vi "Initiate and Generate Time (Multi).vi"(0 "niUsrpRio Sessions":T3[](array[typedef]) {"Daughterboard Clock Rate" format="%#.3pHz"; "FPGA Data Clock Rate" format="%#.3pHz"; "Data Clock Rate" format="%#.3pHz"; "Characterization Data"."Frequencies [Hz]" format="%#_6p"; "EEPROM Characterization Header"."Pointer to Device Data Header" format="%x"; "EEPROM Characterization Header"."Checksum" format="%x"; "Device Data Header"."Pointer to Characterization Data" format="%x"; "Device Data Header"."Checksum" format="%x"; "EEPROM Header"."Pointer to User Header" format="%x"; "EEPROM Header"."Pointer to Factory Header" format="%x"; "EEPROM Header"."Product Code" format="%x"; "EEPROM Header"."Checksum" format="%x"}, 1 "tx channels":T2(array[cluster]) {"tx.coerced configurations"."coerced sample rates" format="%#.3pS/s"; "tx.coerced configurations"."coerced levels" format="%#.3gdBm"; "tx.coerced configurations"."coerced lo frequencies" format="%#.3pHz"; "tx.coerced configurations"."coerced frequencies" format="%#.3pHz"; "tx config"."tone frequency" format="%#.3pHz"; "tx config"."sample rate" format="%#.3pS/s"; "tx config"."rf config 0"."level" format="%#_gdBm"; "tx config"."rf config 0"."lo frequency" format="%#.3pHz"; "tx config"."rf config 0"."frequency" format="%#.3pHz"; "tx config"."rf config 1"."level" format="%#_gdBm"; "tx config"."rf config 1"."lo frequency" format="%#.3pHz"; "tx config"."rf config 1"."frequency" format="%#.3pHz"}, 5 "first iteration":bool, 7 "start trigger time":timestamp, 11 "error in":errorcluster) -> (4 "niUsrpRio Sessions (out)":T3[](array[typedef]) {"Daughterboard Clock Rate" format="%#.3pHz"; "FPGA Data Clock Rate" format="%#.3pHz"; "Data Clock Rate" format="%#.3pHz"; "Characterization Data"."Frequencies [Hz]" format="%#_6p"; "EEPROM Characterization Header"."Pointer to Device Data Header" format="%x"; "EEPROM Characterization Header"."Checksum" format="%x"; "Device Data Header"."Pointer to Characterization Data" format="%x"; "Device Data Header"."Checksum" format="%x"; "EEPROM Header"."Pointer to User Header" format="%x"; "EEPROM Header"."Pointer to Factory Header" format="%x"; "EEPROM Header"."Product Code" format="%x"; "EEPROM Header"."Checksum" format="%x"}, 15 "error out":errorcluster)   [LabVIEW 2015]
doc: "Writes baseband waveform to the device then initiates generation.\n\nVIs that must execute before this VI:\nOpen and Configure.vi\n\n<B>Input Parameters</B>\n\n<B>niUsrpRio Session</B> is the object created by the Open VI and used as the session handle for the USRP RIO design library.\n\n<B>first iteration</B> is used to determine if the device needs to be triggered. If this VI is in a loop, wire the iteration count to Equals Zero and then to this terminal. If this VI is not in a loop, wire a TRUE constant to this this terminal.\n\n<B>start trigger time</B> specifies the absolute time to initiate the start trigger. Only applies when the start trigger is set to Future Event.\n\n<B>error in</B> describes error conditions that occur before this node runs. This input provides standard 'error in' functionality.\n\n<B>Output Parameters</B>\n\n<B>niUsrpRio Session (out)</B> is the niUsrpRio session used in all subsequent USRP RIO design library host VIs.\n\n<B>error out</B> contains error information. This output provides standard 'error out' functionality."
uses:
  <instrlib>/niUsrpRio/Config/v1/Host/Public/niUsrpRio Session.ctl
  <instrlib>/_niInstr/Register Bus/v0/Host/Public/Register Bus Session.ctl
  <instrlib>/_niInstr/Register Bus/v0/Host/Private/Session Data.ctl
  <instrlib>/niUsrpRio/Config/v1/Host/Private/DB Queue Reference.ctl
  <instrlib>/niUsrpRio/Config/v1/Host/Private/Daughterboard Data.ctl
  <instrlib>/niUsrpRio/Config/v1/Host/Private/ATR state data.ctl
  <instrlib>/niUsrpRio/Config/v1/Host/Private/Antenna Configuration.ctl
  <instrlib>/niUsrpRio/Config/v1/Host/Private/CPLD Power Mode.ctl
  <instrlib>/niUsrpRio/Config/v1/Host/Public/EEPROM Header.ctl
  <instrlib>/niUsrpRio/Config/v1/Host/Public/EEPROM Device Data Header.ctl
  <instrlib>/niUsrpRio/Config/v1/Host/Public/EEPROM Characterization Header.ctl
  <instrlib>/niUsrpRio/Config/v1/Host/Public/Characterization Data.ctl
  <instrlib>/niUsrpRio/Config/v1/Host/Public/IQ Imbalance.ctl
  Start Trigger.ctl
  Write Tx Data (I16 multi).vi
  <instrlib>/_niInstr/Register Bus/v0/Host/niInstr Register Bus v0 Host.lvlib
  <instrlib>/niUsrpRio/Config/v1/Host/niUsrpRio Config v1 Host.lvlib
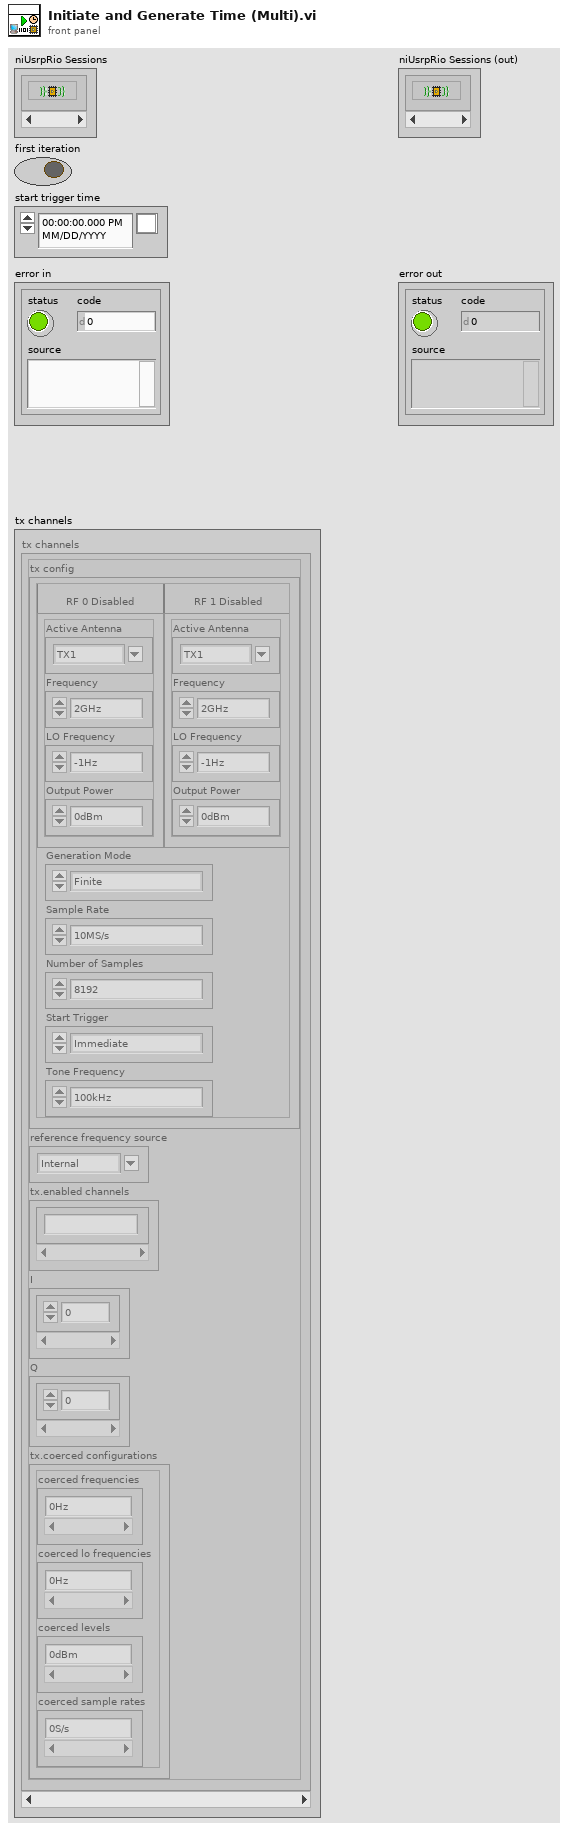
[diagram p1: front panel]
types:
  T1 = typedef "Start Trigger.ctl" = enum8{"Software", "Digital Edge", "Rx Start Trigger", "Tx Start Trigger", "Immediate", "Future Time Event"}
  T2 = cluster{"tx config":cluster{"rf enable 0":bool, "rf config 0":cluster{"antenna":string, "frequency":dbl, "lo frequency":dbl, "level":dbl}, "rf enable 1":bool, "rf config 1":cluster{"antenna":string, "frequency":dbl, "lo frequency":dbl, "level":dbl}, "transfer mode":enum16{"Finite", "Continuous"}, "sample rate":dbl, "number of samples":u32, "start trigger":T1, "tone frequency":dbl}, "reference frequency source":string, "tx.enabled channels":string[], "I":i16[], "Q":i16[], "tx.coerced configurations":cluster{"coerced frequencies":dbl[], "coerced lo frequencies":dbl[], "coerced levels":dbl[], "coerced sample rates":dbl[]}}[]
  T3 = typedef "niUsrpRio Config v1 Host.lvlib/niUsrpRio Session.ctl" = cluster{"FPGA Interface":refnum<k20>, "RIO Interface Number":u32, "Data Clock Rate":u32, "FPGA Data Clock Rate":u32, "Global Settings Register Bus":T4, "Radio 0 Settings Register Bus":T4, "Radio 1 Settings Register Bus":T4, "Radio Settings Bus Semaphore":T5, "DB Queues":T6[], "Characterization Data Valid?":bool, "EEPROM Header":T7, "Device Data Header":T8, "EEPROM Characterization Header":T9, "Characterization Data":T10[], "FPGA Current Version":u32, "FPGA Oldest Compatible Version":u32, "Fixed Logic Current Version":u32, "Fixed Logic Oldest Compatible Version":u32, "FPGA Radio Settings Bus Current Version":u32, "FPGA Radio Settings Bus Oldest Compatible Version":u32, "FPGA Board Config Current Version":u32, "FPGA Board Config Oldest Compatible Version":u32, "Daughterboard Clock Rate":u32}
  T4 = typedef "niInstr Register Bus v0 Host.lvlib/Register Bus Session.ctl" = refnum<queue>
  T5 = typedef "Semaphore RefNum" = refnum<k1>
  T6 = typedef "niUsrpRio Config v1 Host.lvlib/DB Queue Reference.ctl" = refnum<queue>
  T7 = typedef "niUsrpRio Config v1 Host.lvlib/EEPROM Header.ctl" = cluster{"Checksum":u32, "Product Code":u16, "Hardware Current Version":u16, "Hardware Oldest Compatible Version":u16, "EEPROM Map Current Version":u16, "EEPROM Map Oldest Compatible Version":u16, "User Password":string, "Pointer to Factory Header":u32, "Pointer to User Header":u32, "Recommended Interval":u16, "Number of Reserved Bytes":i32, "Number of Daughterboards":u8, "Daughterboard IDs":u16[], "Daughterboard Serial Numbers":string[]}
  T8 = typedef "niUsrpRio Config v1 Host.lvlib/EEPROM Device Data Header.ctl" = cluster{"Checksum":u32, "Number of Channels":u8, "Number of Gain Settings":u16[], "Pointer to Characterization Data":u32[], "Number of Reserved Bytes":i32, "Number of Frequencies":u16[]}
  T9 = typedef "niUsrpRio Config v1 Host.lvlib/EEPROM Characterization Header.ctl" = cluster{"Checksum":u32, "Date":timestamp, "Temperature":sgl, "Misc. Info":string, "Pointer to Device Data Header":u32, "Number of Reserved Bytes":i32}
  T10 = typedef "niUsrpRio Config v1 Host.lvlib/Characterization Data.ctl" = cluster{"Gains[dB]":dbl[], "Frequencies [Hz]":dbl[], "IQ Imbalance Table":T11[], "Measured Gains[dB]":dbl[][]}
  T11 = typedef "niUsrpRio Config v1 Host.lvlib/IQ Imbalance.ctl" = cluster{"Gain Imbalance [linear]":dbl, "Phase Imbalance [radians]":dbl, "Offset":cdb}
  T12 = cluster{"tx config":cluster{"rf enable 0":bool, "rf config 0":cluster{"antenna":string, "frequency":dbl, "lo frequency":dbl, "level":dbl}, "rf enable 1":bool, "rf config 1":cluster{"antenna":string, "frequency":dbl, "lo frequency":dbl, "level":dbl}, "transfer mode":enum16{"Finite", "Continuous"}, "sample rate":dbl, "number of samples":u32, "start trigger":T1, "tone frequency":dbl}, "reference frequency source":string, "tx.enabled channels":string[], "I":i16[], "Q":i16[], "tx.coerced configurations":cluster{"coerced frequencies":dbl[], "coerced lo frequencies":dbl[], "coerced levels":dbl[], "coerced sample rates":dbl[]}}
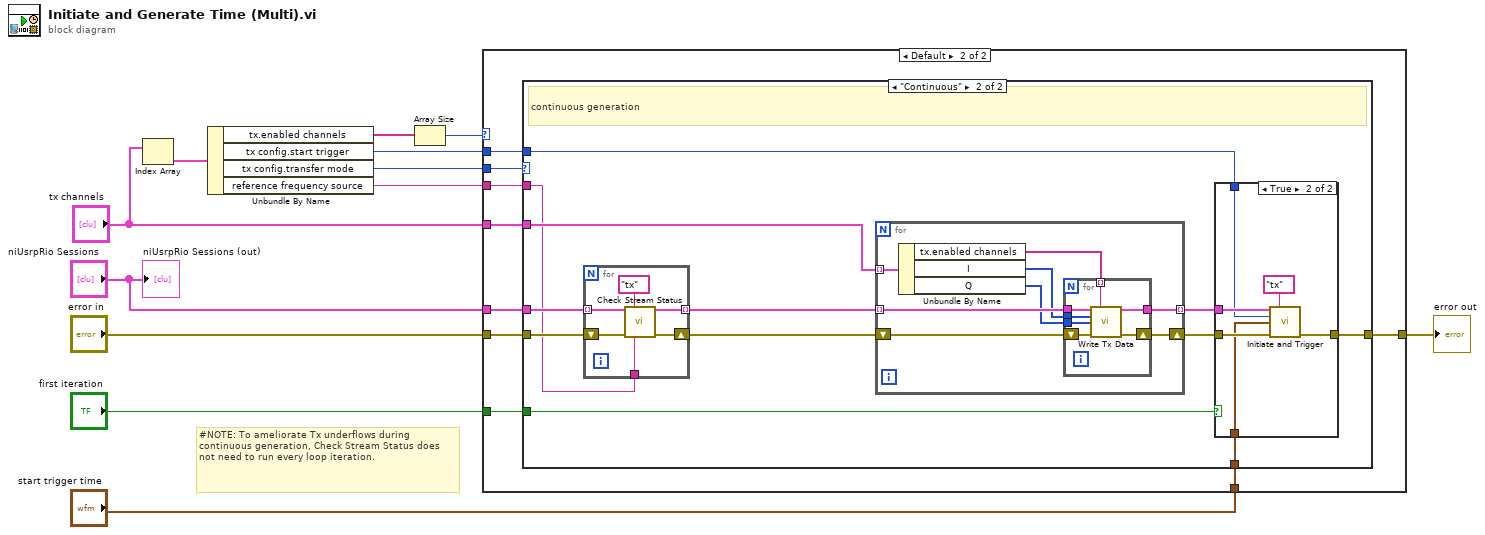
[diagram p0: block diagram]
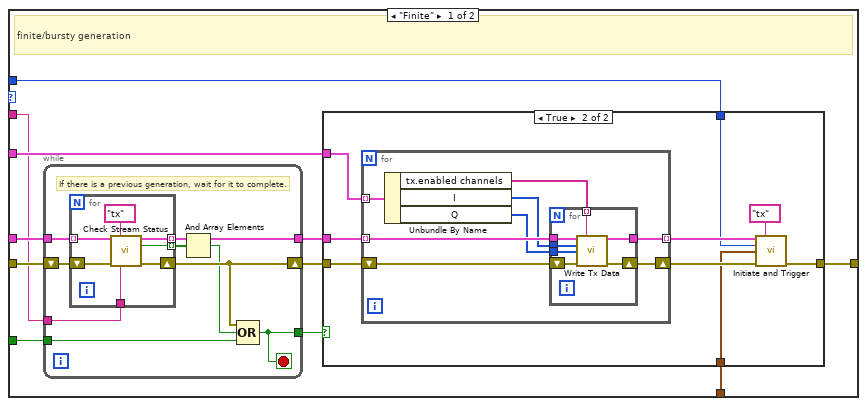
[diagram p3: hidden frame]
diagram:
  # "#NOTE: To ameliorate Tx underflows during continuous generation, Check Stream Status does not need to run every loop iteration."
  n1 = Index Array(array="tx channels") -> (element=w9:T12)  [unwired: 1 in]
  n2 = Unbundle By Name(w9) -> ("tx.enabled channels"=w5:string[], "tx config.start trigger"=w6:T1, "tx config.transfer mode"=w10:enum16{"Finite", "Continuous"}, "reference frequency source"=w7:string)
  n3 = Array Size(array=w5) -> (size(s)=w4:i32)
  n4 = case shown="Default" w4 {
    tunnel: "niUsrpRio Sessions" -> [_ w22]
    tunnel: "error in" -> [w13 w21]
    tunnel: [w13 w20] -> w11
    tunnel: "first iteration" -> [_ w16]
    tunnel: w10 -> [_ w19]
    tunnel: "tx channels" -> [_ w18]
    tunnel: w7 -> [_ w14]
    tunnel: w6 -> [_ w17]
    tunnel: "start trigger time" -> [_ w15]
    frame 0 {
      # "do nothing if there are zero enabled channels"
    }
    frame Default {
      n5 = case shown="\"Continuous\"" w19 {
        tunnel: w22 -> [w24 w79]
        tunnel: w21 -> [w25 w78]
        tunnel: [w33 w86] -> w20
        tunnel: w18 -> [w32 w85]
        tunnel: w17 -> [w31 w84]
        tunnel: w16 -> [w30 w81]
        tunnel: w14 -> [w23 w75]
        tunnel: w15 -> [w28 w80]
        frame "Finite" {
          # "finite/bursty generation"
          n6 = while {
            tunnel: w23 -> [w36]
            shift-right: [w42] -> w27
            shift-left: w25 -> [w39]
            tunnel: w30 -> [w41]
            tunnel: [w34] -> w29
            tunnel: w24 -> [w38]
            tunnel: [w35] -> w26
            stop <- w34 stop-if-true
            # "If there is a previous generation, wait for it to complete."
            n7 = for {
              tunnel: [w49] -> w40 mode=indexing
              shift-right: [w48] -> w42
              shift-left: w39 -> [w47]
              tunnel: w38 -> [w46] mode=indexing
              tunnel: [w45] -> w35 mode=indexing
              tunnel: w36 -> [w43]
              n8 = call "Check Stream Status.vi"("niUsrpRio Session"=w46, "scope"="tx", "error in"=w47, "reference frequency source"=w43) -> ("niUsrpRio Session (out)"=w45:T3, "done"=w49:bool, "error out"=w48:errorcluster)  [unwired: 9 in]
            }
            n9 = And Array Elements(Boolean array=w40) -> (logical AND=w37:bool)
            n10 = Compound Arithmetic op=OR(w42, w37, w41) -> (w34:bool)
          }
          n11 = case shown="True" w29 {
            tunnel: w26 -> [_ w59]
            tunnel: w27 -> [w50 w58]
            tunnel: [w50 w55] -> w33
            tunnel: w32 -> [_ w56]
            tunnel: w31 -> [_ w52]
            tunnel: w28 -> [_ w51]
            frame False {
              # "Do nothing until the previous finite generation finishes before reinitiating."
            }
            frame True {
              n12 = for {
                tunnel: [w64] -> w54 mode=indexing
                tunnel: w59 -> [w66] mode=indexing
                shift-right: [w65] -> w57
                shift-left: w58 -> [w67]
                tunnel: w56 -> [w62] mode=indexing
                n13 = Unbundle By Name(w62) -> ("tx.enabled channels"=w63:string[], "I"=w61:i16[], "Q"=w60:i16[])
                n14 = for {
                  shift-right: [w73] -> w65
                  shift-left: w67 -> [w74]
                  tunnel: w66 -> [w72]
                  tunnel: [w71] -> w64
                  tunnel: w63 -> [w70] mode=indexing
                  tunnel: w61 -> [w69]
                  tunnel: w60 -> [w68]
                  n15 = call-poly "Write Tx Data.vi"("niUsrpRio Session"=w72, "scope"=w70, "I"=w69, "Q"=w68, "error in"=w74) -> ("niUsrpRio Session (out)"=w71:T3, "error out"=w73:errorcluster)  [unwired: 9 in]
                }
              }
              n16 = call "Initiate and Trigger.vi"("niUsrpRio Sessions"=w54, "scope"="tx", "start trigger"=w52, "start trigger time"=w51, "error in"=w57) -> ("error out"=w55:errorcluster)  [unwired: 9 in, 1 out]
            }
          }
        }
        frame "Continuous" {
          # "continuous generation"
          n17 = for {
            shift-right: [w92] -> w76
            shift-left: w78 -> [w91]
            tunnel: w79 -> [w90] mode=indexing
            tunnel: [w89] -> w77 mode=indexing
            tunnel: w75 -> [w87]
            n18 = call "Check Stream Status.vi"("niUsrpRio Session"=w90, "scope"="tx", "error in"=w91, "reference frequency source"=w87) -> ("niUsrpRio Session (out)"=w89:T3, "error out"=w92:errorcluster)  [unwired: 9 in, 1 out]
          }
          n19 = for {
            tunnel: [w104] -> w82 mode=indexing
            tunnel: w77 -> [w106] mode=indexing
            shift-right: [w105] -> w83
            shift-left: w76 -> [w107]
            tunnel: w85 -> [w102] mode=indexing
            n20 = Unbundle By Name(w102) -> ("tx.enabled channels"=w103:string[], "I"=w101:i16[], "Q"=w100:i16[])
            n21 = for {
              shift-right: [w113] -> w105
              shift-left: w107 -> [w114]
              tunnel: w106 -> [w112]
              tunnel: [w111] -> w104
              tunnel: w103 -> [w110] mode=indexing
              tunnel: w101 -> [w109]
              tunnel: w100 -> [w108]
              n22 = call-poly "Write Tx Data.vi"("niUsrpRio Session"=w112, "scope"=w110, "I"=w109, "Q"=w108, "error in"=w114) -> ("niUsrpRio Session (out)"=w111:T3, "error out"=w113:errorcluster)  [unwired: 9 in]
            }
          }
          n23 = case shown="True" w81 {
            tunnel: [w93 w98] -> w86
            tunnel: w84 -> [_ w97]
            tunnel: w83 -> [w93 w96]
            tunnel: w82 -> [_ w99]
            tunnel: w80 -> [_ w94]
            frame False {
              # "Only initiate on first iteration."
            }
            frame True {
              n24 = call "Initiate and Trigger.vi"("niUsrpRio Sessions"=w99, "scope"="tx", "start trigger"=w97, "start trigger time"=w94, "error in"=w96) -> ("error out"=w98:errorcluster)  [unwired: 9 in, 1 out]
            }
          }
        }
      }
    }
  }
  "error out" <- w11
  "niUsrpRio Sessions (out)" <- "niUsrpRio Sessions"
